vi "Config-Read Key (Boolean).vi"(0 "configuration file path":path, 2 "section":string="General", 7 "key":string="CFTS Run Mode", 9 "default":bool, 11 "error in (no error)":errorcluster) -> (4 "file path":path, 8 "found?":bool, 10 "value":bool, 15 "error out":errorcluster)   [LabVIEW 2020]
uses:
  <vilib>/Utility/config.llb/Read Key (Boolean).vi
  <vilib>/Utility/config.llb/NI_LVConfig.lvlib
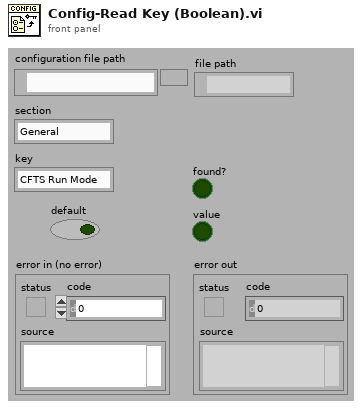
[diagram p1: front panel]
types:
  T1 = typedef "NI_LVConfig.lvlib/Config Data RefNum.ctl" = refnum<k1>
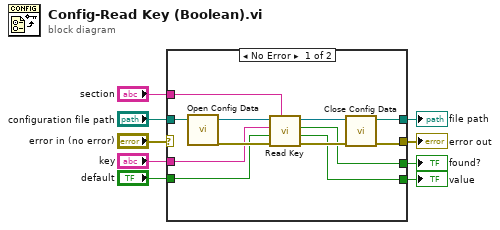
[diagram p0: block diagram]
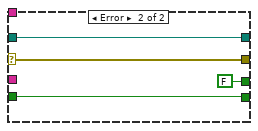
[diagram p2: hidden frame]
diagram:
  n1 = case shown="No Error" "error in (no error)" {
    selector: "error in (no error)" -> [_ w25]
    tunnel: [w19 w25] -> w9
    tunnel: [w16 w22] -> w7
    tunnel: "default" -> [w15 w22]
    tunnel: "key" -> [w14 _]
    tunnel: "section" -> [w13 _]
    tunnel: "configuration file path" -> [w12 w24]
    tunnel: [w11 w24] -> w2
    tunnel: [w10 FALSE ("found?")] -> w1
    frame No Error {
      n2 = call <vilib>:"Open Config Data.vi"("configuration file path"=w12) -> ("error out"=w21:errorcluster, "refnum"=w20:T1)  [unwired: 8 in, 1 out]
      n3 = call-poly <vilib>:"Read Key.vi"("section"=w13, "error in (no error)"=w21, "default value"=w15, "key"=w14, "refnum"=w20) -> ("error out"=w18:errorcluster, "value"=w16:bool, "found?"=w10:bool, "refnum out"=w17:T1)  [unwired: 3 in]
      n4 = call <vilib>:"Close Config Data.vi"("error in (no error)"=w18, "refnum"=w17) -> ("error out"=w19:errorcluster, "file path"=w11:path)  [unwired: 8 in]
    }
    frame Error {
    }
  }
  "error out" <- w9
  "value" <- w7
  "file path" <- w2
  "found?" <- w1
